vi "CLD3 FGV Timer Solution 2.vi"(8 "Error In":errorcluster, 10 "Time Target (s)":dbl=4.0, 11 "Timer Mode":T1) -> (0 "Error Out":errorcluster, 2 "Has Time Elapsed":bool, 3 "Elapsed Time (s.ss)":dbl)   [LabVIEW 2018]
doc: "CLD 3 Exercise"
uses:
  CLD3 FGV Mode.ctl
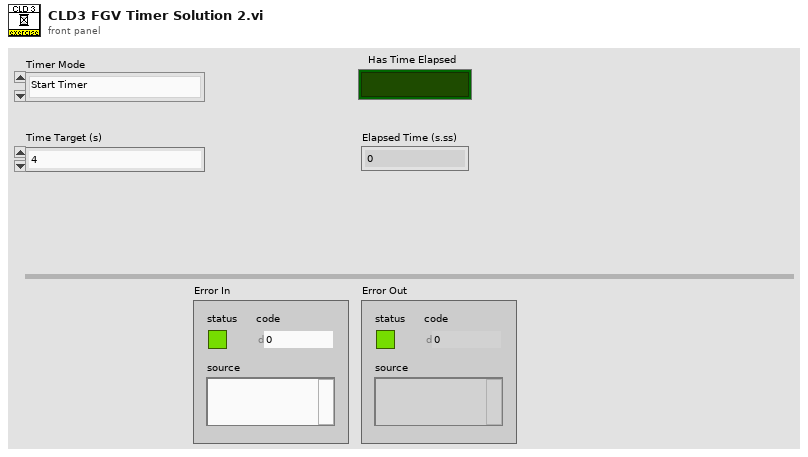
[diagram p1: front panel]
types:
  T1 = typedef "CLD3 FGV Mode.ctl" = enum16{"Start Timer", "Read Time", "Pause", "Resume", "Update Time Target (s)"}
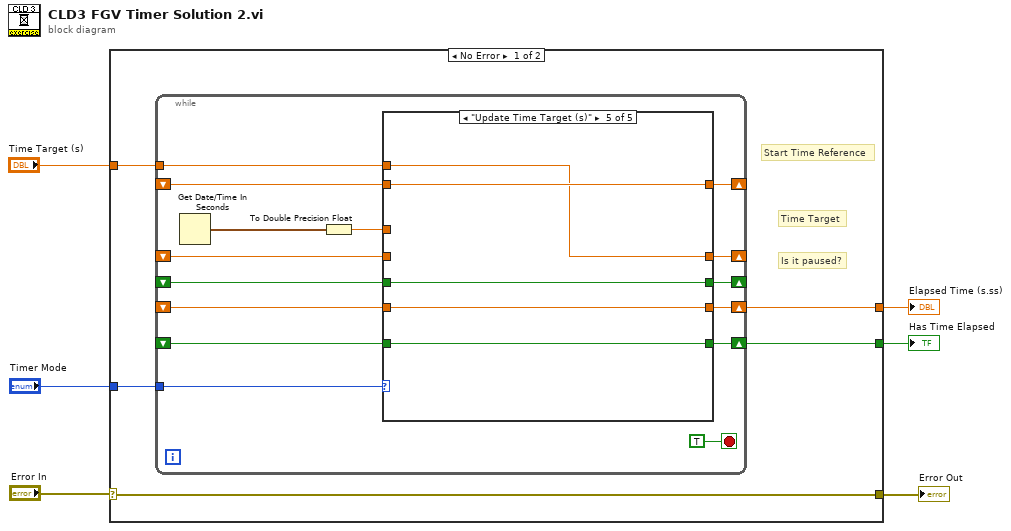
[diagram p0: block diagram]
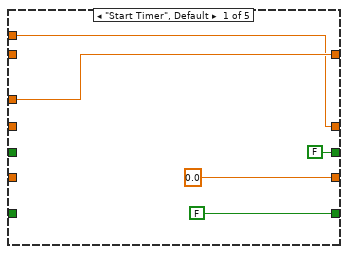
[diagram p2: hidden frame]
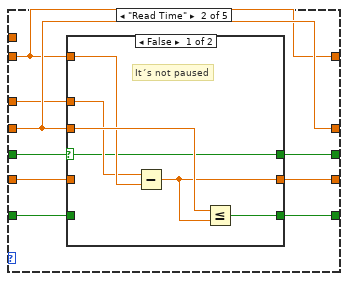
[diagram p3: hidden frame]
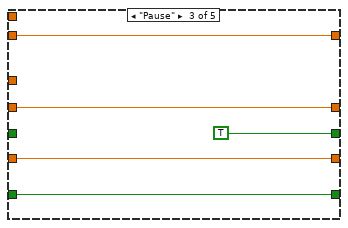
[diagram p5: hidden frame]
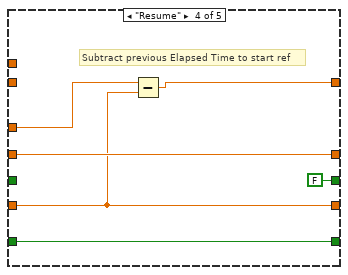
[diagram p6: hidden frame]
diagram:
  n1 = case shown="No Error" "Error In" {
    selector: "Error In" -> [w8 w66]
    tunnel: "Timer Mode" -> [w11 _]
    tunnel: [w10 _] -> w5
    tunnel: [w9 _] -> w4
    tunnel: [w8 w66] -> w2
    tunnel: "Time Target (s)" -> [w7 _]
    frame No Error {
      # "Is it paused?"
      # "Time Target"
      # "Start Time Reference"
      n2 = while {
        tunnel: w11 -> [w26]
        shift-right: [w25] -> _
        shift-left: _ -> [w21]
        shift-right: [w23] -> _
        shift-left: _ -> [w20]
        shift-right: [w22] -> w10
        shift-left: _ -> [w18]
        shift-right: [w19] -> w9
        shift-left: _ -> [w15]
        shift-right: [w14] -> _
        shift-left: _ -> [w13]
        tunnel: w7 -> [w12]
        stop <- TRUE stop-if-true
        n3 = Get Date/Time In Seconds() -> (seconds since 1Jan1904=w17:timestamp)
        n4 = To Double Precision Float(number=w17) -> (double precision float=w16:dbl)
        n5 = case shown="\"Update Time Target (s)\"" w26 {
          tunnel: [w29 w37 w51 w57 w65] -> w25
          tunnel: [w27 w40 w54 w60 w61] -> w23
          tunnel: [0.0 ("Time Target (s)") w39 w53 w58 w63] -> w22
          tunnel: w21 -> [_ w37 w51 _ w65]
          tunnel: w20 -> [_ w40 w54 w60 _]
          tunnel: [FALSE w38 w52 w59 w64] -> w19
          tunnel: w18 -> [_ w33 w53 w58 w63]
          tunnel: w16 -> [w29 w36 _ w56 _]
          tunnel: w15 -> [_ w34 w52 w59 w64]
          tunnel: [FALSE w32 TRUE FALSE w62] -> w14
          tunnel: w13 -> [_ w35 _ _ w62]
          tunnel: w12 -> [w27 _ _ _ w61]
          frame "Start Timer", Default {
          }
          frame "Read Time" {
            n6 = case shown="False" w35 {
              selector: w35 -> [w41 w47]
              tunnel: w40 -> [w46 _]
              tunnel: [w45 w48] -> w39
              tunnel: [w44 w49] -> w38
              tunnel: w37 -> [w43 _]
              tunnel: w36 -> [w42 _]
              tunnel: w34 -> [_ w49]
              tunnel: w33 -> [_ w48]
              tunnel: [w41 w47] -> w32
              frame False {
                # "It´s not paused"
                n7 = Subtract(x=w42, y=w43) -> (x-y=w45:dbl)
                n8 = Less Or Equal?(x=w46, y=w45) -> (x <= y?=w44:bool)
              }
              frame True {
              }
            }
          }
          frame "Pause" {
          }
          frame "Resume" {
            # "Subtract previous Elapsed Time to start ref"
            n9 = Subtract(x=w56, y=w58) -> (x-y=w57:dbl)
          }
          frame "Update Time Target (s)" {
          }
        }
      }
    }
    frame Error {
    }
  }
  "Error Out" <- w2
  "Elapsed Time (s.ss)" <- w5
  "Has Time Elapsed" <- w4
